vi "Read Guardian List.vi"(8 "error in (no error)":errorcluster, 11 "Guardian in":refnum<class "Guardian.lvclass">) -> (0 "error out":errorcluster, 2 "TALOS.lvlib:Classes.lvlib:Guardian List.lvclass":refnum<class "Guardian List.lvclass">, 3 "Guardian out":refnum<class "Guardian.lvclass">)   [LabVIEW 2026, in "TALOS.lvlib" / "Guardian.lvlib" / "Guardian.lvclass"]
uses:
  Guardian.lvclass
  Classes/Guardian List/Guardian List.lvclass
  Guardian.lvclass/Guardian.ctl
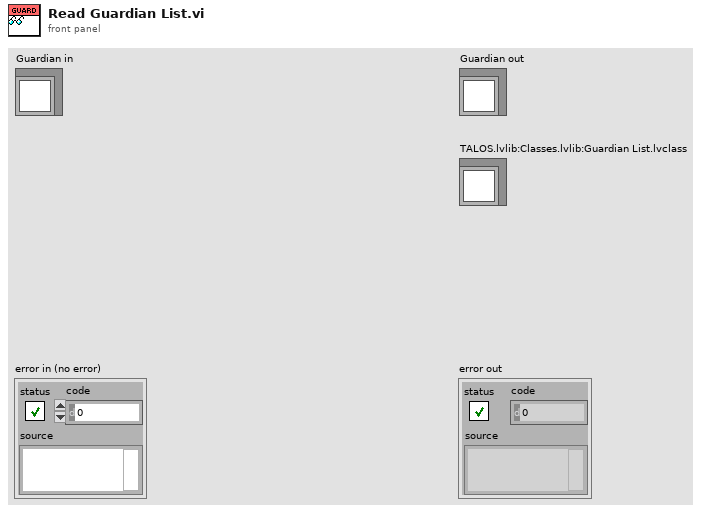
[diagram p1: front panel]
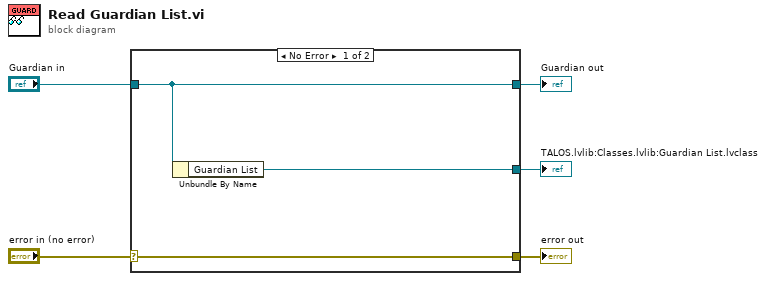
[diagram p0: block diagram]
diagram:
  n1 = case shown="No Error" "error in (no error)" {
    selector: "error in (no error)" -> [w8 w9]
    tunnel: [w8 w9] -> w4
    tunnel: [w7 w10] -> w2
    tunnel: "Guardian in" -> [w7 w10]
    tunnel: [w6 _] -> w1
    frame No Error {
      n2 = Unbundle By Name(w7) -> ("Guardian List"=w6:refnum<class "Guardian List.lvclass">)
    }
    frame Error {
    }
  }
  "error out" <- w4
  "Guardian out" <- w2
  "TALOS.lvlib:Classes.lvlib:Guardian List.lvclass" <- w1
